vi "Build Experiment.vi"(0 "object in":refnum<class "Experiment.lvclass">, 1 "Triggering":T2, 2 "Levels":dbl[](array[numeric]), 3 "Ramp In Settings":T1, 4 "Number of Images at each Level":u16, 5 "error in (no error)":errorcluster) -> (14 "object out":refnum<class "Experiment.lvclass">, 19 "error out":errorcluster)   [LabVIEW 2021, in "Experiment.lvclass"]
uses:
  Experiment.lvclass
  Experiment.lvclass/Experiment.ctl
panel:
  # "DIO0 Pulses at the same time as DIO1,2 and 3 +-offset"
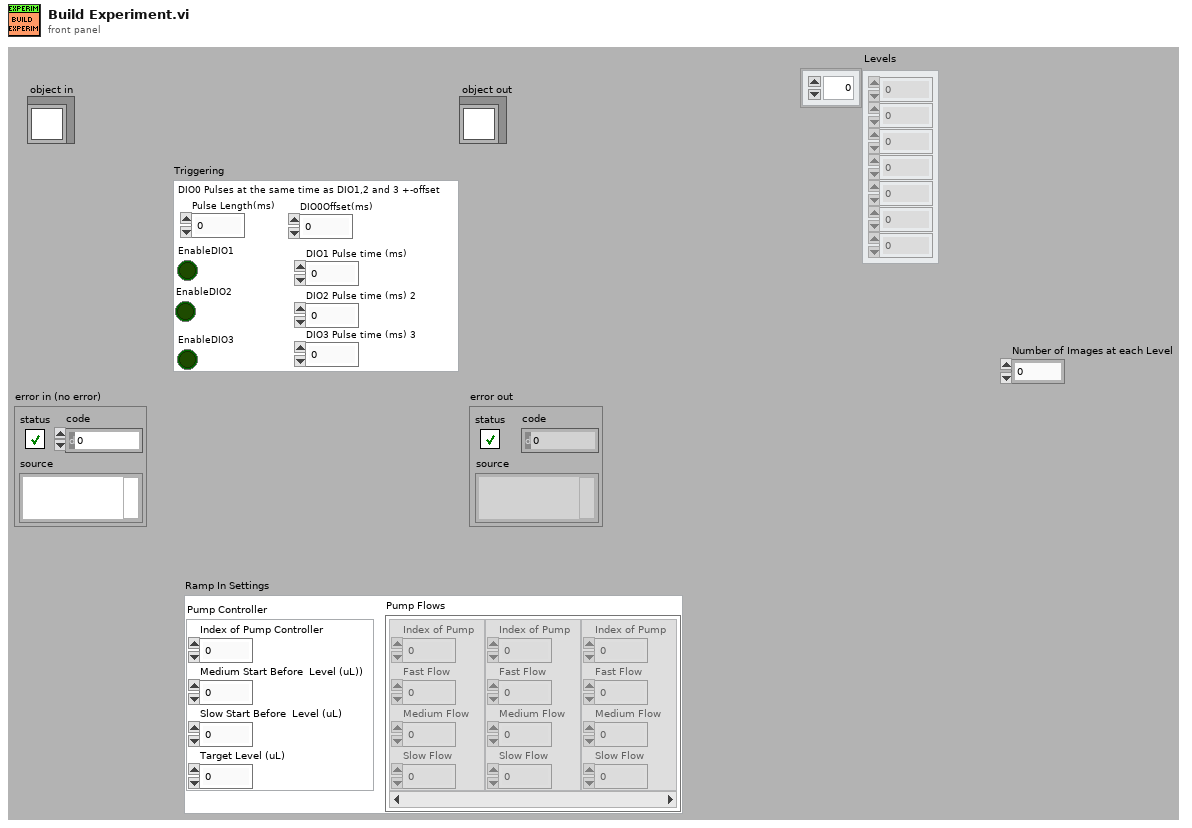
[diagram p1: front panel]
types:
  T1 = cluster{"Pump Controller":cluster{"Index of Pump Controller":u8, "Medium Start Before  Level (uL))":dbl, "Slow Start Before  Level (uL)":dbl, "Target Level (uL)":dbl}, "Pump Flows":cluster{"Index of Pump":u8, "Fast Flow":dbl, "Medium Flow":dbl, "Slow Flow":dbl}[]}
  T2 = cluster{"Pulse Length(ms)":dbl, "DIO0Offset(ms)":dbl, "DIO1 Pulse time (ms)":dbl, "DIO2 Pulse time (ms) 2":dbl, "DIO3 Pulse time (ms) 3":dbl, "EnableDIO3":bool, "EnableDIO2":bool, "EnableDIO1":bool}
  T3 = cluster{"Ramp In Settings":cluster{"Pump Controller":cluster{"Index of Pump Controller":u8, "Medium Start Before  Level (uL))":dbl, "Slow Start Before  Level (uL)":dbl, "Target Level (uL)":dbl}, "Pump Flows":cluster{"Index of Pump":u8, "Fast Flow":dbl, "Medium Flow":dbl, "Slow Flow":dbl}[]}, bool}
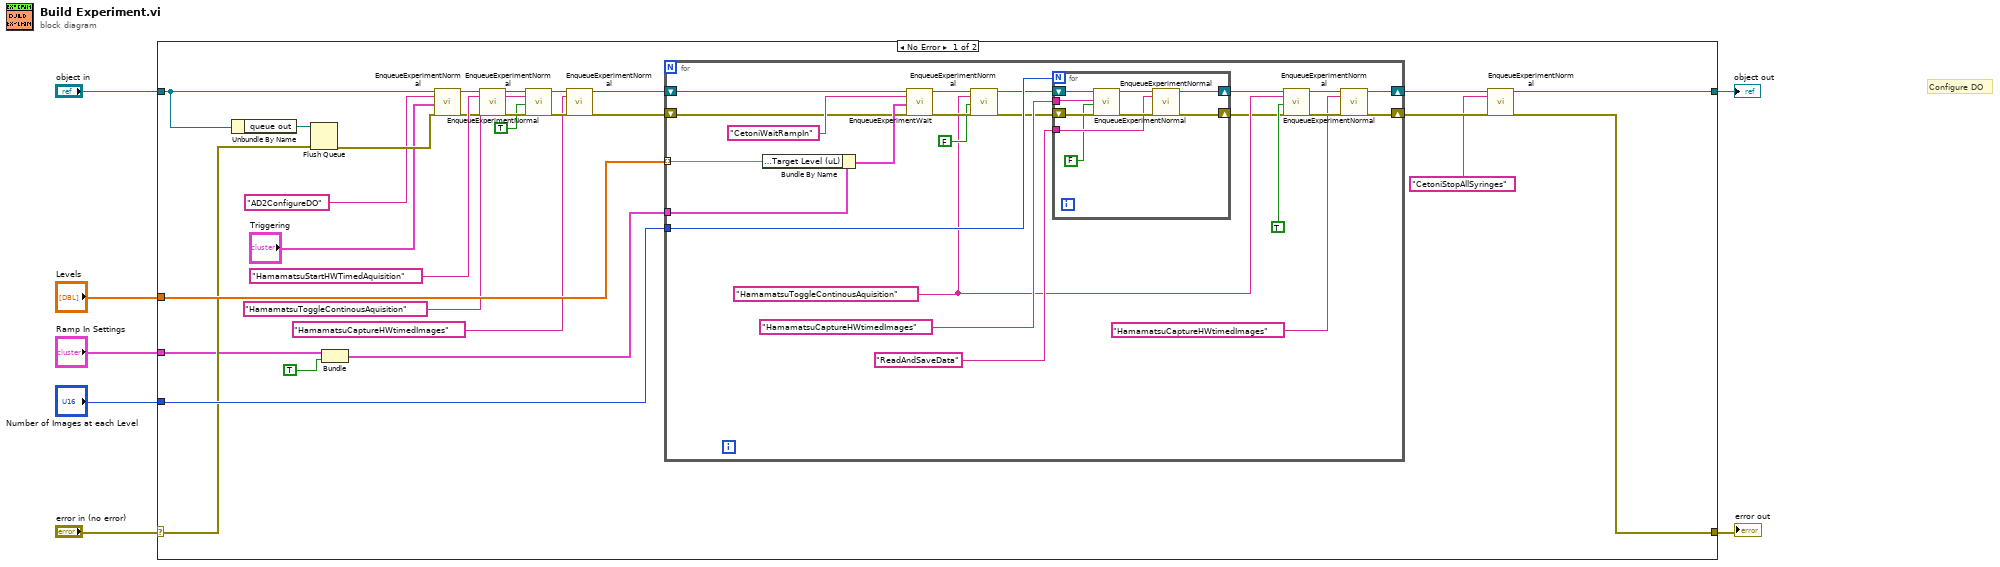
[diagram p0: block diagram]
diagram:
  # "Configure DO"
  n1 = case shown="No Error" "error in (no error)" {
    selector: "error in (no error)" -> [w20 w69]
    tunnel: [w21 w69] -> w6
    tunnel: [w22 w68] -> w4
    tunnel: "object in" -> [w33 w68]
    tunnel: "Levels" -> [w34 _]
    tunnel: "Number of Images at each Level" -> [w26 _]
    tunnel: "Ramp In Settings" -> [w17 _]
    frame No Error {
      n2 = Unbundle By Name(w33) -> ("queue out"=w35:refnum<queue>)
      n3 = Flush Queue(queue=w35, error in (no error)=w20) -> (error out=w32:errorcluster)  [unwired: 2 out]
      n4 = Bundle("Ramp In Settings"=w17, TRUE) -> (w18:T3)  [unwired: 1 in]
      n5 = call-dynamic "EnqueueExperimentNormal.vi"("object in"=w33, "Message"="AD2ConfigureDO", "Message Data"="Triggering", "error in (no error)"=w32) -> ("object out"=w29:refnum<class "Experiment.lvclass">, "error out"=w27:errorcluster)  [unwired: 14 in]
      n6 = call-dynamic "EnqueueExperimentNormal.vi"("object in"=w29, "Message"="HamamatsuStartHWTimedAquisition", "error in (no error)"=w27) -> ("object out"=w14:refnum<class "Experiment.lvclass">, "error out"=w12:errorcluster)  [unwired: 15 in]
      n7 = call-dynamic "EnqueueExperimentNormal.vi"("object in"=w14, "Message"="HamamatsuToggleContinousAquisition", "Message Data"=TRUE, "error in (no error)"=w12) -> ("object out"=w16:refnum<class "Experiment.lvclass">, "error out"=w15:errorcluster)  [unwired: 14 in]
      n8 = call-dynamic "EnqueueExperimentNormal.vi"("object in"=w16, "Message"="HamamatsuCaptureHWtimedImages", "error in (no error)"=w15) -> ("object out"=w13:refnum<class "Experiment.lvclass">, "error out"=w11:errorcluster)  [unwired: 15 in]
      n9 = for {
        tunnel: w34 -> [w57] mode=indexing
        tunnel: w18 -> [w58]
        shift-right: [w39] -> w25
        shift-left: w13 -> [w56]
        tunnel: w26 -> [w52]
        shift-right: [w37] -> w24
        shift-left: w11 -> [w53]
        w43 = "HamamatsuToggleContinousAquisition" ("Message")
        n10 = Bundle By Name(cluster=w58, "Ramp In Settings.Pump Controller.Target Level (uL)"=w57) -> (w54:T3)
        n11 = call-dynamic "EnqueueExperimentWait.vi"("object in"=w56, "Message"="CetoniWaitRampIn", "Message Data"=w54, "error in (no error)"=w53) -> ("object out"=w49:refnum<class "Experiment.lvclass">, "error out"=w47:errorcluster)  [unwired: 14 in]
        n12 = call-dynamic "EnqueueExperimentNormal.vi"("object in"=w49, "Message"=w43, "Message Data"=FALSE, "error in (no error)"=w47) -> ("object out"=w48:refnum<class "Experiment.lvclass">, "error out"=w46:errorcluster)  [unwired: 14 in]
        n13 = for {
          N: w52 -> [_]
          shift-right: [w64] -> w44
          shift-left: w48 -> [w67]
          shift-right: [w62] -> w41
          shift-left: w46 -> [w66]
          tunnel: "HamamatsuCaptureHWtimedImages" ("Message") -> [w61]
          tunnel: "ReadAndSaveData" ("Message") -> [w60]
          n14 = call-dynamic "EnqueueExperimentNormal.vi"("object in"=w67, "Message"=w61, "Message Data"=FALSE, "error in (no error)"=w66) -> ("object out"=w65:refnum<class "Experiment.lvclass">, "error out"=w63:errorcluster)  [unwired: 14 in]
          n15 = call-dynamic "EnqueueExperimentNormal.vi"("object in"=w65, "Message"=w60, "error in (no error)"=w63) -> ("object out"=w64:refnum<class "Experiment.lvclass">, "error out"=w62:errorcluster)  [unwired: 15 in]
        }
        n16 = call-dynamic "EnqueueExperimentNormal.vi"("object in"=w44, "Message"=w43, "Message Data"=TRUE, "error in (no error)"=w41) -> ("object out"=w40:refnum<class "Experiment.lvclass">, "error out"=w38:errorcluster)  [unwired: 14 in]
        n17 = call-dynamic "EnqueueExperimentNormal.vi"("object in"=w40, "Message"="HamamatsuCaptureHWtimedImages", "error in (no error)"=w38) -> ("object out"=w39:refnum<class "Experiment.lvclass">, "error out"=w37:errorcluster)  [unwired: 15 in]
      }
      n18 = call-dynamic "EnqueueExperimentNormal.vi"("object in"=w25, "Message"="CetoniStopAllSyringes", "error in (no error)"=w24) -> ("object out"=w22:refnum<class "Experiment.lvclass">, "error out"=w21:errorcluster)  [unwired: 15 in]
    }
    frame Error {
    }
  }
  "error out" <- w6
  "object out" <- w4
